vi "GetHelp.vi"(11 "DiffVI in":refnum<class "DiffVI.lvclass">) -> (2 "Help":string, 3 "DiffVI out":refnum<class "DiffVI.lvclass">)   [LabVIEW 2015, in "DiffVI.lvclass"]
uses:
  DiffVI.lvclass
panel:
  in  "Help":string="LabVIEWCLI -OperationName DiffVI -OldVI <path of old VI> -NewVI <path of new VI> -OutputDir <path of output directory>"
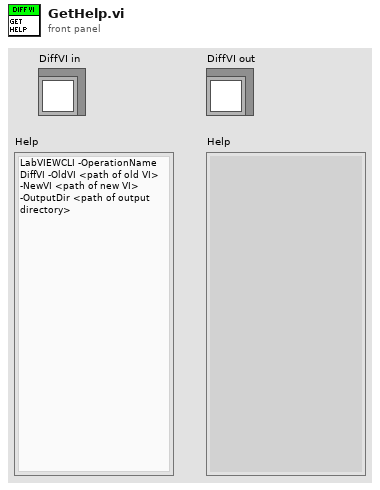
[diagram p1: front panel]
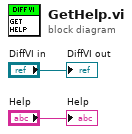
[diagram p0: block diagram]
diagram:
  "DiffVI out" <- "DiffVI in"
  "Help" <- "Help"
